vi "New Entity.vi"(7 "Entity Type":refnum<class "Entity.lvclass">, 8 "error in (no error)":errorcluster, 11 "Entity Manager in":refnum<class "Entity Manager.lvclass">) -> (0 "error out":errorcluster, 2 "Entity":refnum<class "Entity.lvclass">, 3 "Entity Manager out":refnum<class "Entity Manager.lvclass">)   [LabVIEW 2020, in "Conditum.lvlib" / "Entity Manager.lvclass"]
uses:
  Entity Manager.lvclass
  Entity/Entity.lvclass
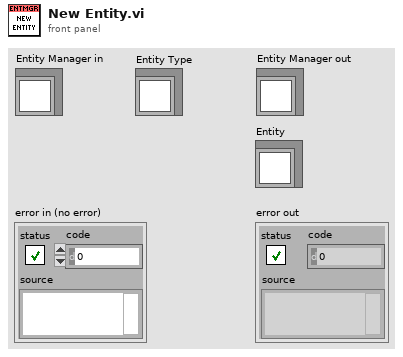
[diagram p1: front panel]
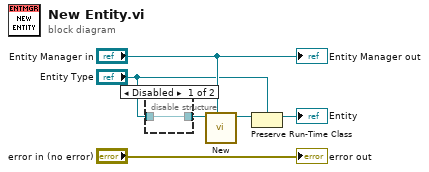
[diagram p0: block diagram]
diagram:
  n1 = disable-structure shown="Disabled" {
    disable-tunnel: "Entity Type" -> [w7 _]
    disable-tunnel: [w7 _] -> w5
    frame Disabled {
    }
    frame Enabled {
    }
  }
  n2 = call "New.vi"("Entity Manager"="Entity Manager in", "Entity in"=w5) -> ("Entity out"=w3:refnum<class "Entity.lvclass">)  [unwired: 9 in]
  n3 = Preserve Run-Time Class(object in=w3, 2:"Entity Type") -> (object out=→"Entity":refnum<class "Entity.lvclass">)  [unwired: 1 in, 1 out]
  "error out" <- "error in (no error)"
  "Entity Manager out" <- "Entity Manager in"
